vi "Home Page.vi"() -> ()   [LabVIEW 2020]
uses:
  ctl/Generate Report.ctl
  ctl/Add Data Source.ctl
  ctl/Create Datasets.ctl
panel:
  in  "stop":bool
  in  "Add Datasets":T1
  in  "Add Data Source":T2
  in  "Generate Report":T3
  # "HOME PAGE"
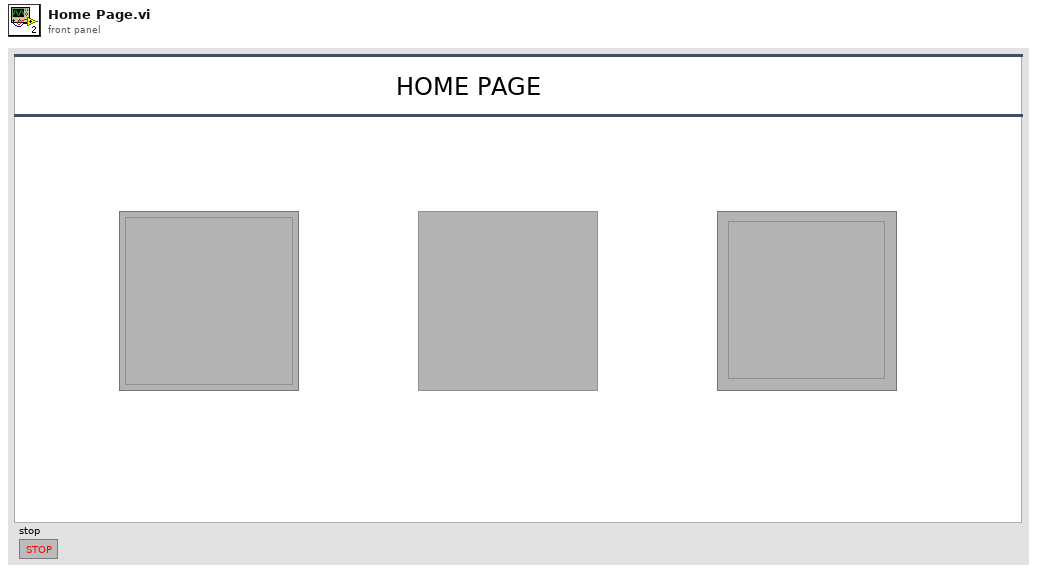
[diagram p1: front panel]
types:
  T1 = typedef "Create Datasets.ctl" = bool
  T2 = typedef "Add Data Source.ctl" = bool
  T3 = typedef "Generate Report.ctl" = bool
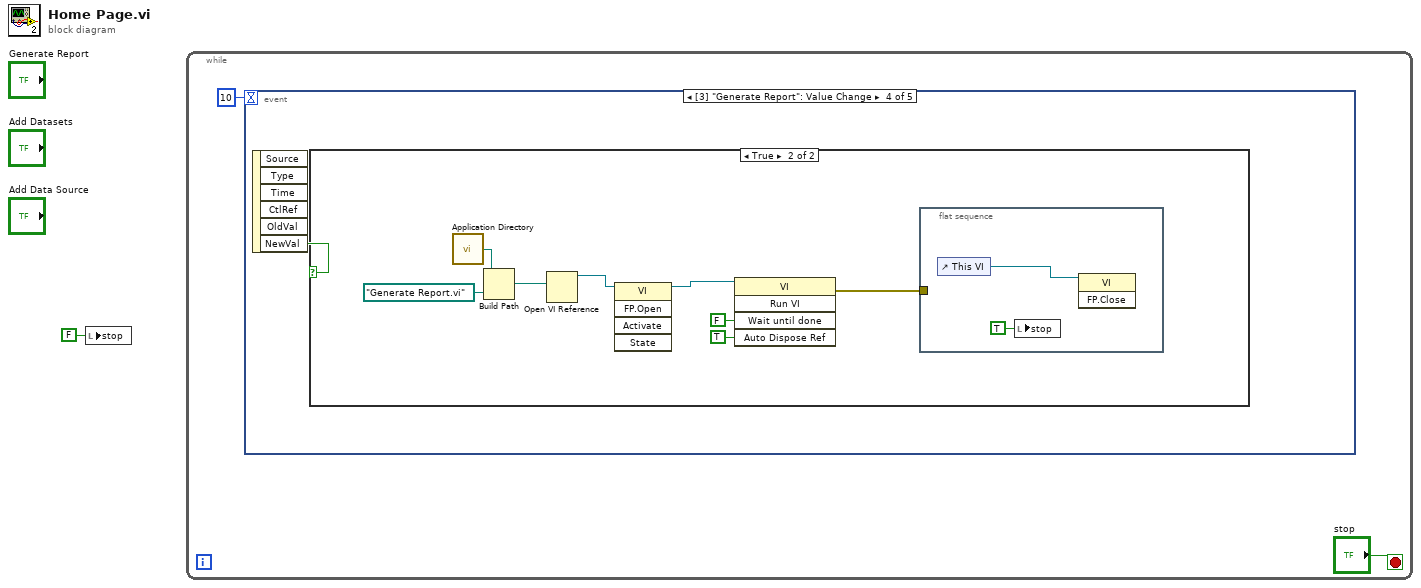
[diagram p0: block diagram]
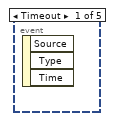
[diagram p2: hidden frame]
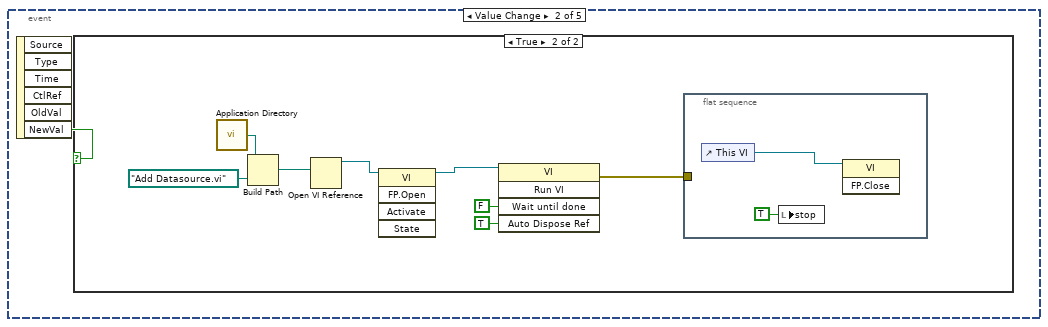
[diagram p3: hidden frame]
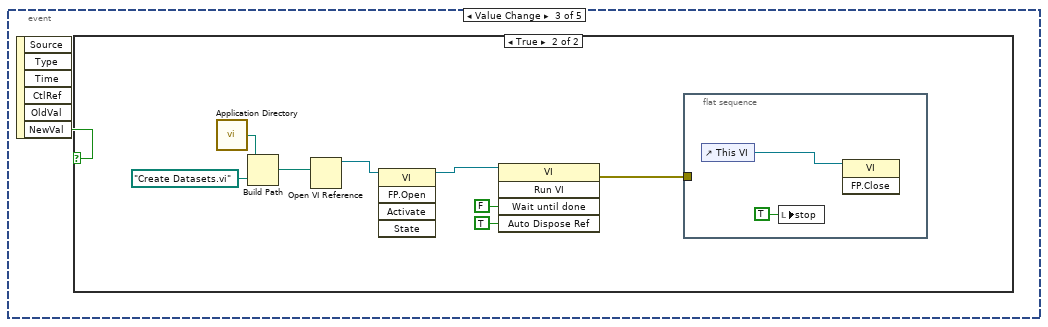
[diagram p5: hidden frame]
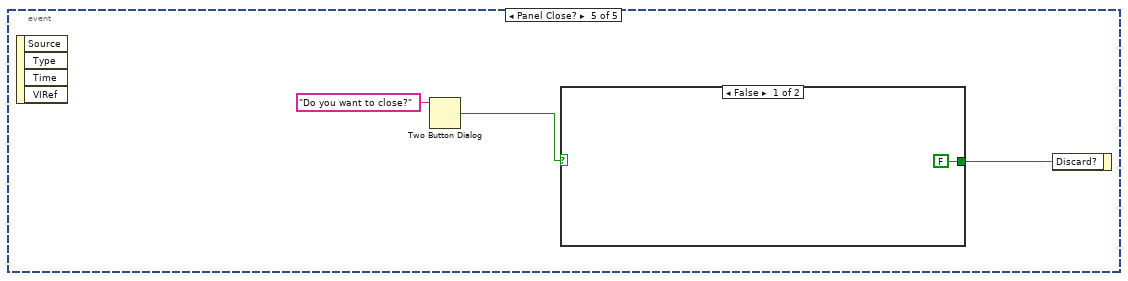
[diagram p8: hidden frame]
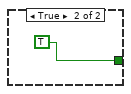
[diagram p9: hidden frame]
diagram:
  n1 = local write "stop"(FALSE ("stop")) -> ()
  n2 = while {
    stop <- "stop" stop-if-true
    n3 = event shown="[3] \"Generate Report\": Value Change" {
      selector: _ -> [_ _ _ _ _]
      dyn-events: _ -> [_ _ _ _ _]
      timeout: 10 -> [_ _ _ _ _]
      event Timeout {
        n4 = event-data() -> ()  [unwired: 1 in, 3 out]
      }
      event Value Change {
        n5 = event-data() -> ("NewVal"=w4:T2)  [unwired: 1 in, 5 out]
        n6 = case shown="True" w4 {
          frame False {
          }
          frame True {
            n7 = call <vilib>:"Application Directory.vi"() -> ("Application Directory"=w12:path)
            n8 = Build Path(base path=w12, name or relative path=path "Add Datasource.vi") -> (appended path=w10:path)
            n9 = Open VI Reference(vi path=w10) -> (vi reference=w9:refnum<vi>)  [unwired: 5 in, 1 out]
            n10 = invoke class="VI" method="FP.Open"(reference=w9) -> (reference out=w8:refnum<vi>)  [unwired: 4 in, 4 out]
            n11 = invoke class="VI" method="Run VI"(reference=w8, "Wait until done"=FALSE ("Wait Until Done"), "Auto Dispose Ref"=TRUE ("Auto Dispose Reference")) -> (error out=w6:errorcluster)  [unwired: 2 in, 4 out]
            n12 = flat-sequence {
              tunnel: w6 -> [_]
              frame #0 {
                n13 = control-ref of="This VI"() -> (w14:refnum<vi>)
                n14 = local write "stop"(TRUE ("stop")) -> ()
                n15 = invoke class="VI" method="FP.Close"(reference=w14) -> ()  [unwired: 2 in, 3 out]
              }
            }
          }
        }
      }
      event Value Change {
        n16 = event-data() -> ("NewVal"=w15:T1)  [unwired: 1 in, 5 out]
        n17 = case shown="True" w15 {
          frame False {
          }
          frame True {
            n18 = call <vilib>:"Application Directory.vi"() -> ("Application Directory"=w23:path)
            n19 = Build Path(base path=w23, name or relative path=path "Create Datasets.vi") -> (appended path=w21:path)
            n20 = Open VI Reference(vi path=w21) -> (vi reference=w20:refnum<vi>)  [unwired: 5 in, 1 out]
            n21 = invoke class="VI" method="FP.Open"(reference=w20) -> (reference out=w19:refnum<vi>)  [unwired: 4 in, 4 out]
            n22 = invoke class="VI" method="Run VI"(reference=w19, "Wait until done"=FALSE ("Wait Until Done"), "Auto Dispose Ref"=TRUE ("Auto Dispose Reference")) -> (error out=w17:errorcluster)  [unwired: 2 in, 4 out]
            n23 = flat-sequence {
              tunnel: w17 -> [_]
              frame #0 {
                n24 = control-ref of="This VI"() -> (w25:refnum<vi>)
                n25 = local write "stop"(TRUE ("stop")) -> ()
                n26 = invoke class="VI" method="FP.Close"(reference=w25) -> ()  [unwired: 2 in, 3 out]
              }
            }
          }
        }
      }
      event Value Change {
        n27 = event-data() -> ("NewVal"=w26:T3)  [unwired: 1 in, 5 out]
        n28 = case shown="True" w26 {
          frame False {
          }
          frame True {
            n29 = call <vilib>:"Application Directory.vi"() -> ("Application Directory"=w34:path)
            n30 = Build Path(base path=w34, name or relative path=path "Generate Report.vi") -> (appended path=w32:path)
            n31 = Open VI Reference(vi path=w32) -> (vi reference=w31:refnum<vi>)  [unwired: 5 in, 1 out]
            n32 = invoke class="VI" method="FP.Open"(reference=w31) -> (reference out=w30:refnum<vi>)  [unwired: 4 in, 4 out]
            n33 = invoke class="VI" method="Run VI"(reference=w30, "Wait until done"=FALSE ("Wait Until Done"), "Auto Dispose Ref"=TRUE ("Auto Dispose Reference")) -> (error out=w28:errorcluster)  [unwired: 2 in, 4 out]
            n34 = flat-sequence {
              tunnel: w28 -> [_]
              frame #0 {
                n35 = control-ref of="This VI"() -> (w36:refnum<vi>)
                n36 = local write "stop"(TRUE ("stop")) -> ()
                n37 = invoke class="VI" method="FP.Close"(reference=w36) -> ()  [unwired: 2 in, 3 out]
              }
            }
          }
        }
      }
      event Panel Close? {
        n38 = event-data() -> ()  [unwired: 1 in, 4 out]
        n39 = Two Button Dialog(message="Do you want to close?") -> (T button?=w37:bool)  [unwired: 2 in]
        n40 = case shown="False" w37 {
          tunnel: [FALSE ("Discard?") TRUE ("Discard?")] -> w39
          frame False {
          }
          frame True {
          }
        }
        n41 = event-data("Discard?"=w39) -> ()  [unwired: 1 in, 1 out]
      }
    }
  }
